vi "JTAG F-RAM.vi"(0 "Function":T1(ring), 5 "Opcode":u16(ring)=6 items=["WREN (Set WrEn Latch) 0x06"=6, "WRDI (Wr Disable) 0x04"=4, "RDSR (Rd Status Reg) 0x05"=5, "WRSR (Wr Status Reg) 0x01"=1, "READ (Rd Memory Data) 0x03"=3, "FSTRD (Fast Rd) 0x0B"=11, "WRITE (Wr Memory Data) 0x02"=2, "SLEEP (Sleep Mode) 0xB9"=185, "RDID (Rd Device ID) 0x9F"=159, "SNR (Rd Serial Number) 0xC3"=195], 7 "Address":u16 format="%04x", 9 "Value":u8 format="%02x", 11 "error in (no error)":errorcluster, 12 "Blocksize":u16 format="%03d", 13 "Block Write Data":u8[](array[numeric]) format="%02x") -> (4 "Read Value":u8 format="%.0x", 6 "Block Read Data":u16[](array[numeric]) format="%02x", 15 "error out":errorcluster)   [LabVIEW 2010]
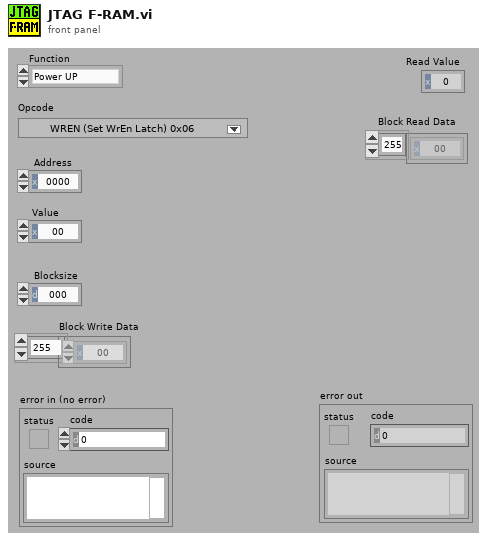
[diagram p1: front panel]
types:
  T1 = enum16{"Power UP", "Power DN", "Read Single", "Write Single", "Read Block", "Write Block", "Read SR", "Write SR", "Send Opcode"}
  T2 = enum8{"PORT_OUT", "PORT_SEL", "PORT_RES_EN", "READ_PORT", "PORT_DIR", "SET_LCM", "PLUTO_WRITE_SINGLE", "PLUTO_READ_SINGLE", "PLUTO_WRITE_MASK", "STIM_POWER_UP", "STIM_POWER_DN", "SATURN_WRITE_SINGLE", "SATURN_READ_SINGLE", "SATURN_WRITE_BLOCK", "SATURN_READ_BLOCK", "SATURN_WRITE_MASK", "MICS_POWER_UP", "MICS_POWER_DN", "MICS_WRITE_SINGLE", "MICS_READ_SINGLE", "MICS_WRITE_BLOCK", "MICS_READ_BLOCK", "MICS_WRITE_MASK", "MEM_POWER_UP", "MEM_POWER_DN", "MEM_WRITE_SINGLE", "MEM_READ_SINGLE", "MEM_WRITE_BLOCK", "MEM_READ_BLOCK", "MEM_WRITE_MASK", "MEM_WRITE_SR", "MEM_READ_SR", "MEM_OPCODE", "INIT_VARIABLES", "DCO -> 1 MHz", "DCO -> 8 MHz", "START_STIM_CLK", "STOP_STIM_CLK", "PULSE_STIM_CLK", "PULSE_STIM_SCK", "SINGLE_ADC12", "SINGLE_ADC12_REPEAT", "MULTI_ADC12", "MULTI_ADC12_REPEAT", "Disable_ADC12", "READ_IO_VARIABLES"}
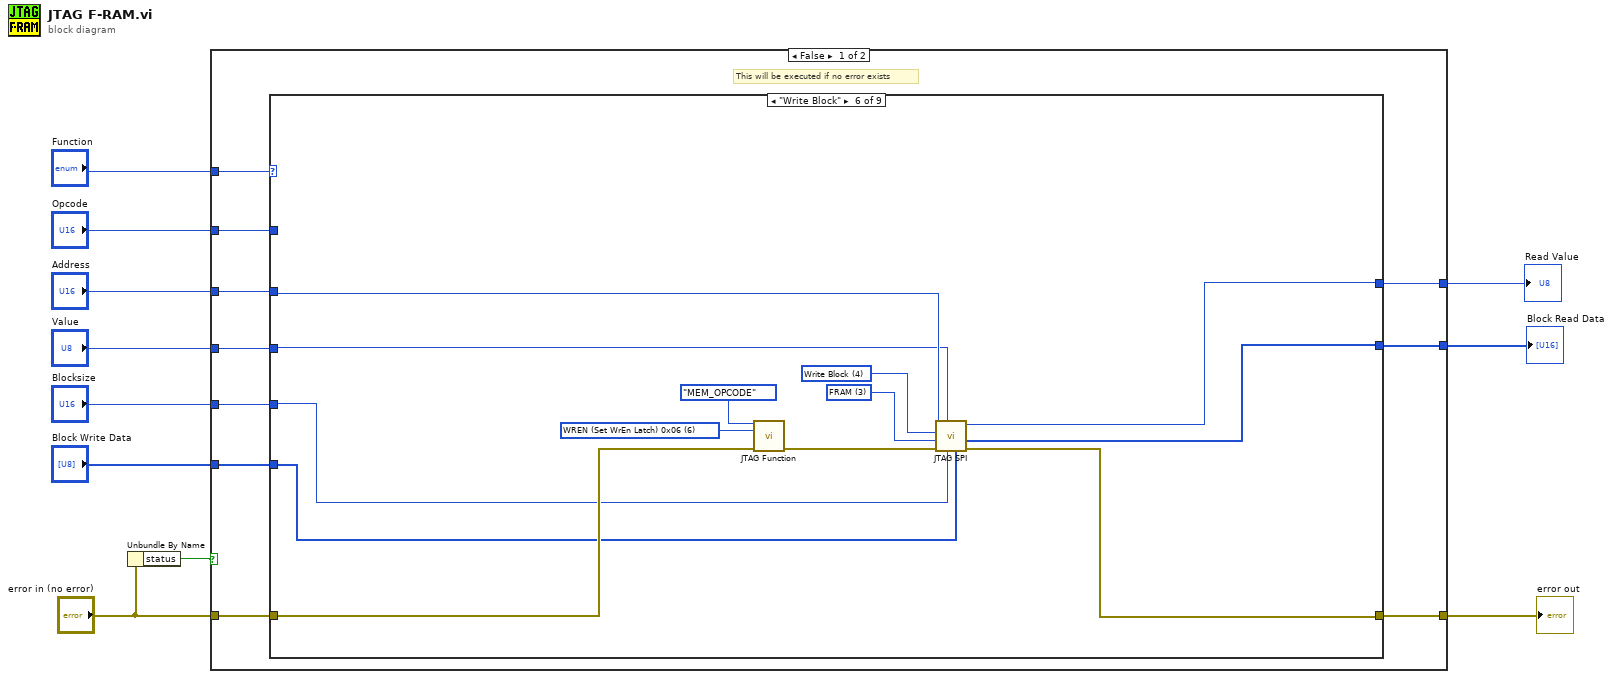
[diagram p0: block diagram]
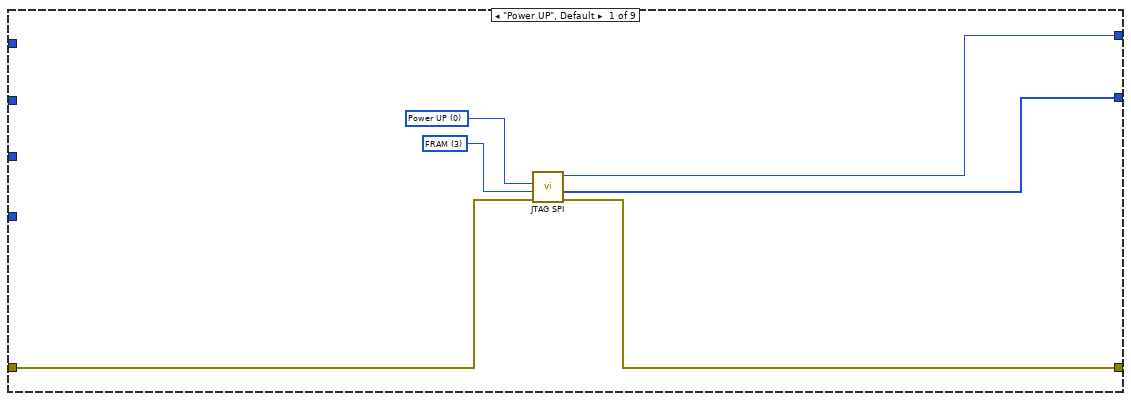
[diagram p2: hidden frame]
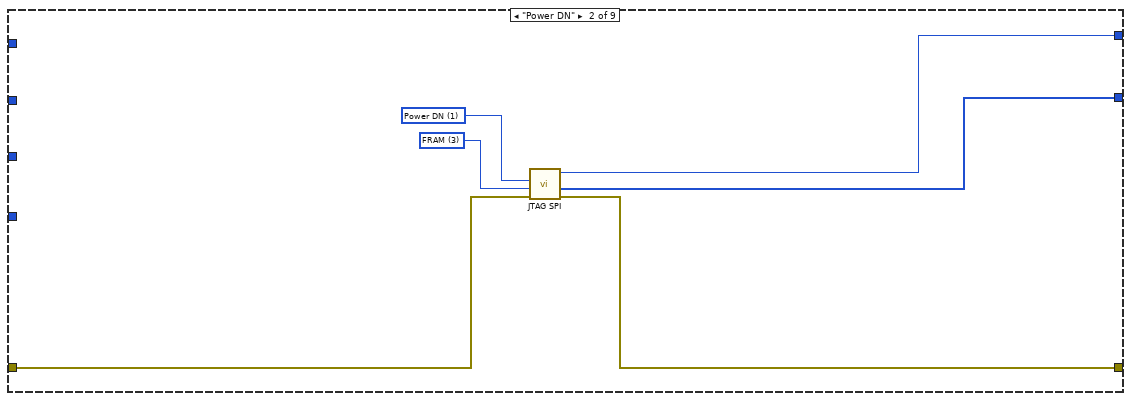
[diagram p3: hidden frame]
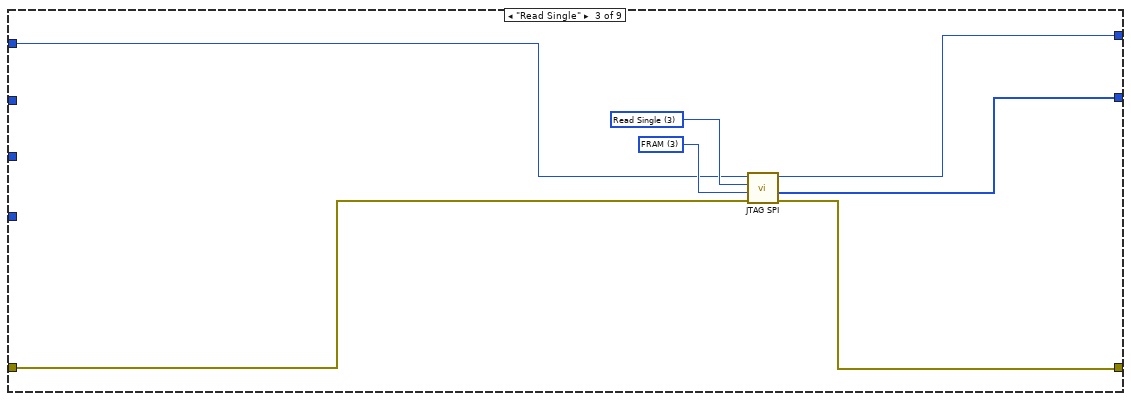
[diagram p4: hidden frame]
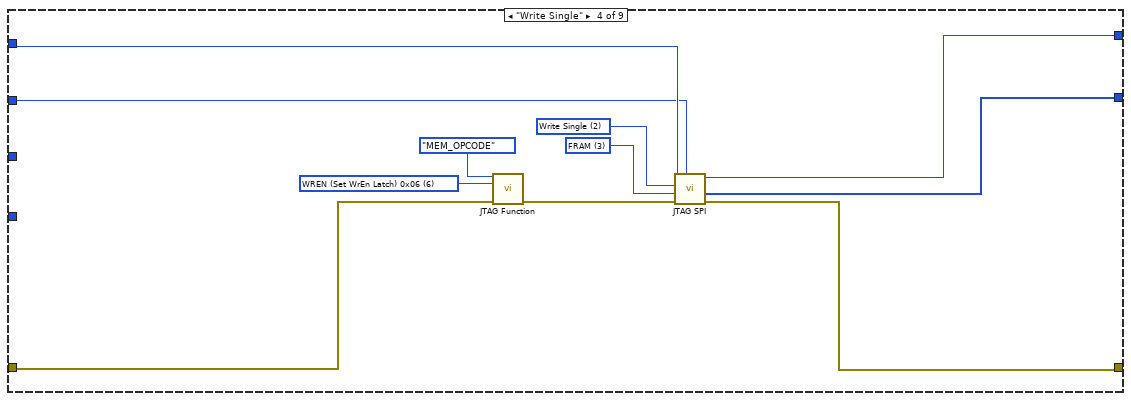
[diagram p5: hidden frame]
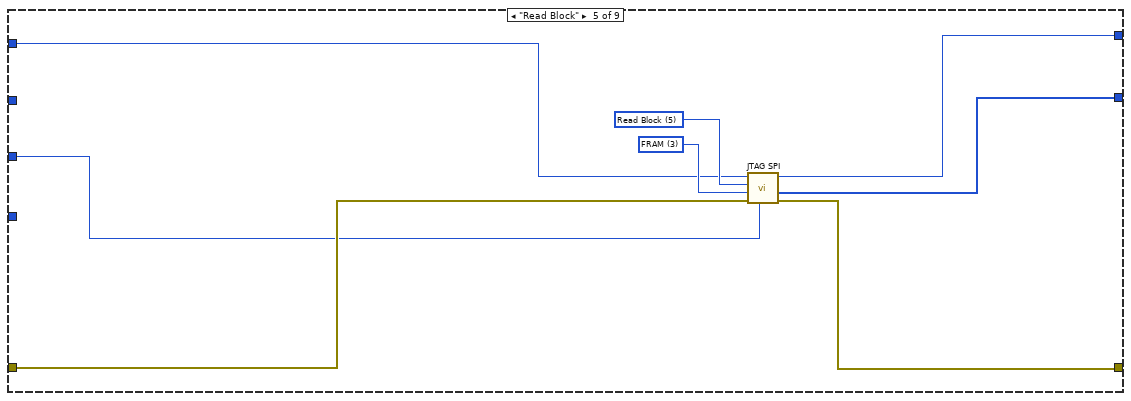
[diagram p6: hidden frame]
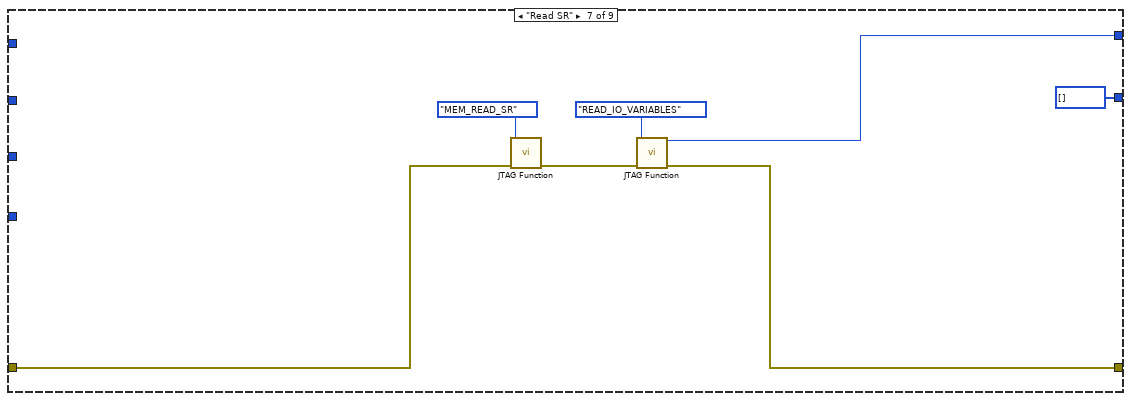
[diagram p7: hidden frame]
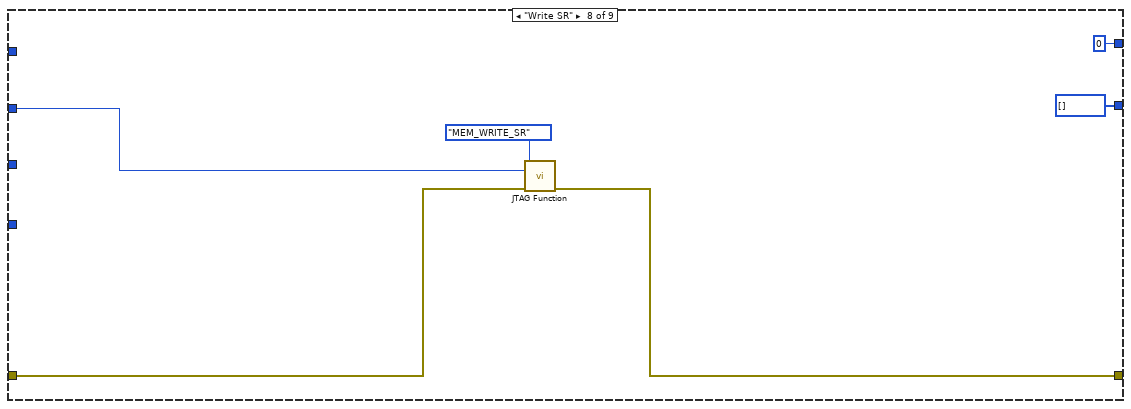
[diagram p8: hidden frame]
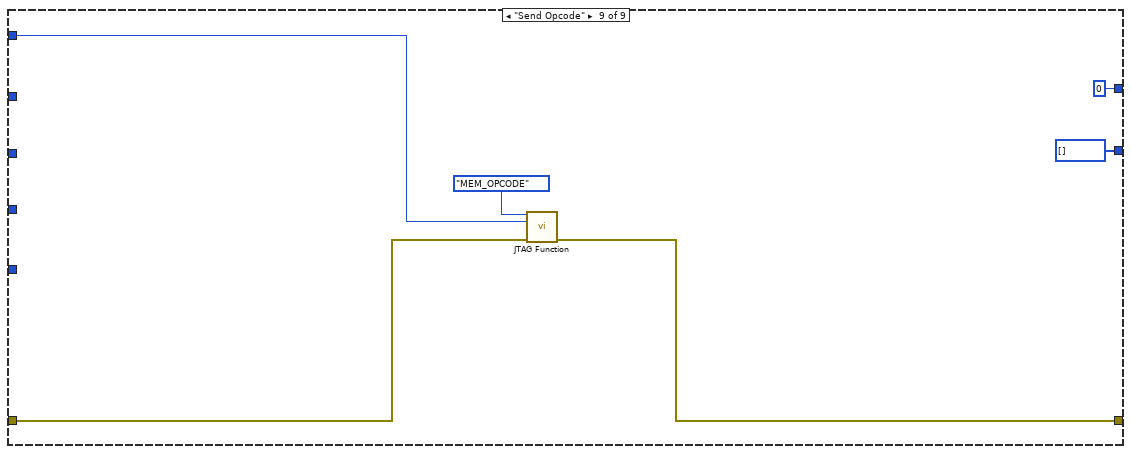
[diagram p9: hidden frame]
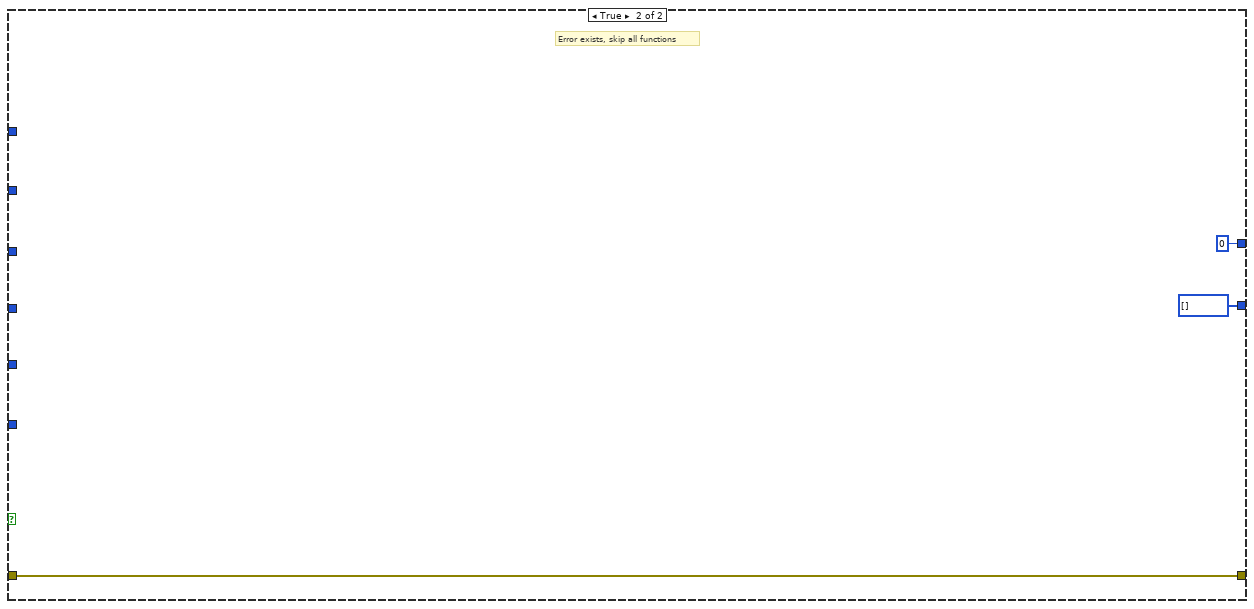
[diagram p10: hidden frame]
diagram:
  n1 = Unbundle By Name("error in (no error)") -> ("status"=w10:bool)
  n2 = case shown="False" w10 {
    tunnel: [w20 w94] -> w11
    tunnel: "error in (no error)" -> [w21 w94]
    tunnel: "Function" -> [w19 _]
    tunnel: "Address" -> [w18 _]
    tunnel: [w17 u16 0 ("ARG 7")] -> w6
    tunnel: "Value" -> [w16 _]
    tunnel: "Blocksize" -> [w15 _]
    tunnel: [w14 u16[] [] ("Block Read Data")] -> w3
    tunnel: "Block Write Data" -> [w13 _]
    tunnel: "Opcode" -> [w12 _]
    frame False {
      # "This will be executed if no error exists"
      n3 = case shown="\"Write Block\"" w19 {
        tunnel: w21 -> [w27 w31 w38 w45 w57 w65 w78 w84 w88]
        tunnel: [w26 w30 w37 w48 w55 w64 w75 w83 w87] -> w20
        tunnel: w18 -> [_ _ w36 w49 w56 w67 _ _ _]
        tunnel: [w23 w28 w35 w47 w54 w62 w73 u16 0 ("ARG 7") u16 0 ("ARG 7")] -> w17
        tunnel: w16 -> [_ _ _ w46 _ w66 _ w82 _]
        tunnel: w15 -> [_ _ _ _ w53 w61 _ _ _]
        tunnel: [w22 w29 w34 w41 w52 w63 u16[] [] ("Block Read Data") u16[] [] ("Block Read Data") u16[] [] ("Block Read Data")] -> w14
        tunnel: w13 -> [_ _ _ _ _ w60 _ _ _]
        tunnel: w12 -> [_ _ _ _ _ _ _ _ w86]
        frame "Power UP", Default {
          w24 = u16 3 items=["Power ASIC", "Stim ASIC", "MICS Radio", "FRAM"] ("Target")
          w25 = u16 0 items=["Power UP", "Power DN", "Write Single", "Read Single", "Write Block", "Read Block", "Write Masked", "Test Value"] ("Function")
          n4 = call "JTAG SPI.vi"("error in (no error)"=w27, "Target"=w24, "Function"=w25) -> ("error out"=w26:errorcluster, "Block Read Data"=w22:u16[], "Read Value"=w23:u8)  [unwired: 5 in, 1 out]
        }
        frame "Power DN" {
          w32 = u16 3 items=["Power ASIC", "Stim ASIC", "MICS Radio", "FRAM"] ("Target")
          w33 = u16 1 items=["Power UP", "Power DN", "Write Single", "Read Single", "Write Block", "Read Block", "Write Masked", "Test Value"] ("Function")
          n5 = call "JTAG SPI.vi"("error in (no error)"=w31, "Target"=w32, "Function"=w33) -> ("error out"=w30:errorcluster, "Block Read Data"=w29:u16[], "Read Value"=w28:u8)  [unwired: 5 in, 1 out]
        }
        frame "Read Single" {
          w39 = u16 3 items=["Power ASIC", "Stim ASIC", "MICS Radio", "FRAM"] ("Target")
          w40 = u16 3 items=["Power UP", "Power DN", "Write Single", "Read Single", "Write Block", "Read Block", "Write Masked", "Test Value"] ("Function")
          n6 = call "JTAG SPI.vi"("error in (no error)"=w38, "Target"=w39, "Function"=w40, "Address"=w36) -> ("error out"=w37:errorcluster, "Block Read Data"=w34:u16[], "Read Value"=w35:u8)  [unwired: 4 in, 1 out]
        }
        frame "Write Single" {
          w42 = u16 6 items=["WREN (Set WrEn Latch) 0x06"=6, "WRDI (Wr Disable) 0x04"=4, "RDSR (Rd Status Reg) 0x05"=5, "WRSR (Wr Status Reg) 0x01"=1, "READ (Rd Memory Data) 0x03"=3, "FSTRD (Fast Rd) 0x0B"=11, "WRITE (Wr Memory Data) 0x02"=2, "SLEEP (Sleep Mode) 0xB9"=185, "RDID (Rd Device ID) 0x9F"=159, "SNR (Rd Serial Number) 0xC3"=195] ("Opcode")
          w50 = u16 3 items=["Power ASIC", "Stim ASIC", "MICS Radio", "FRAM"] ("Target")
          w51 = u16 2 items=["Power UP", "Power DN", "Write Single", "Read Single", "Write Block", "Read Block", "Write Masked", "Test Value"] ("Function")
          n7 = call "JTAG Function.vi"("Enum"=T2."MEM_OPCODE", "ARG 1"=w42, "error in (no error)"=w45) -> ("error out"=w44:errorcluster)  [unwired: 10 in, 2 out]
          n8 = call "JTAG SPI.vi"("Value"=w46, "error in (no error)"=w44, "Target"=w50, "Function"=w51, "Address"=w49) -> ("error out"=w48:errorcluster, "Block Read Data"=w41:u16[], "Read Value"=w47:u8)  [unwired: 3 in, 1 out]
        }
        frame "Read Block" {
          w58 = u16 3 items=["Power ASIC", "Stim ASIC", "MICS Radio", "FRAM"] ("Target")
          w59 = u16 5 items=["Power UP", "Power DN", "Write Single", "Read Single", "Write Block", "Read Block", "Write Masked", "Test Value"] ("Function")
          n9 = call "JTAG SPI.vi"("Blocksize"=w53, "error in (no error)"=w57, "Target"=w58, "Function"=w59, "Address"=w56) -> ("error out"=w55:errorcluster, "Block Read Data"=w52:u16[], "Read Value"=w54:u8)  [unwired: 3 in, 1 out]
        }
        frame "Write Block" {
          w68 = u16 6 items=["WREN (Set WrEn Latch) 0x06"=6, "WRDI (Wr Disable) 0x04"=4, "RDSR (Rd Status Reg) 0x05"=5, "WRSR (Wr Status Reg) 0x01"=1, "READ (Rd Memory Data) 0x03"=3, "FSTRD (Fast Rd) 0x0B"=11, "WRITE (Wr Memory Data) 0x02"=2, "SLEEP (Sleep Mode) 0xB9"=185, "RDID (Rd Device ID) 0x9F"=159, "SNR (Rd Serial Number) 0xC3"=195] ("Opcode")
          w71 = u16 3 items=["Power ASIC", "Stim ASIC", "MICS Radio", "FRAM"] ("Target")
          w72 = u16 4 items=["Power UP", "Power DN", "Write Single", "Read Single", "Write Block", "Read Block", "Write Masked", "Test Value"] ("Function")
          n10 = call "JTAG Function.vi"("Enum"=T2."MEM_OPCODE", "ARG 1"=w68, "error in (no error)"=w65) -> ("error out"=w70:errorcluster)  [unwired: 10 in, 2 out]
          n11 = call "JTAG SPI.vi"("Block Write Data"=w60, "Blocksize"=w61, "Value"=w66, "error in (no error)"=w70, "Target"=w71, "Function"=w72, "Address"=w67) -> ("error out"=w64:errorcluster, "Block Read Data"=w63:u16[], "Read Value"=w62:u8)  [unwired: 1 in, 1 out]
        }
        frame "Read SR" {
          n12 = call "JTAG Function.vi"("Enum"=T2."MEM_READ_SR", "error in (no error)"=w78) -> ("error out"=w76:errorcluster)  [unwired: 11 in, 2 out]
          n13 = call "JTAG Function.vi"("Enum"=T2."READ_IO_VARIABLES", "error in (no error)"=w76) -> ("ARG 7"=w73:u16, "error out"=w75:errorcluster)  [unwired: 11 in, 1 out]
        }
        frame "Write SR" {
          n14 = call "JTAG Function.vi"("Enum"=T2."MEM_WRITE_SR", "ARG 1"=w82, "error in (no error)"=w84) -> ("error out"=w83:errorcluster)  [unwired: 10 in, 2 out]
        }
        frame "Send Opcode" {
          n15 = call "JTAG Function.vi"("Enum"=T2."MEM_OPCODE", "ARG 1"=w86, "error in (no error)"=w88) -> ("error out"=w87:errorcluster)  [unwired: 10 in, 2 out]
        }
      }
    }
    frame True {
      # "Error exists, skip all functions"
    }
  }
  "error out" <- w11
  "Read Value" <- w6
  "Block Read Data" <- w3
